vi "CmdExe.Command Line Output to Log text.vi"(11 "CmdLineOut":T1) -> (3 "Log Text":string)   [LabVIEW 2024]
uses:
  CmdExe.Command Line Output Info.ctl
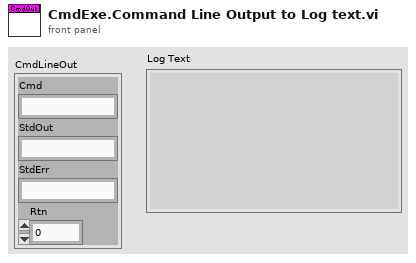
[diagram p1: front panel]
types:
  T1 = typedef "CmdExe.Command Line Output Info.ctl" = cluster{"Cmd":string, "StdOut":string, "StdErr":string, "Rtn":i32}
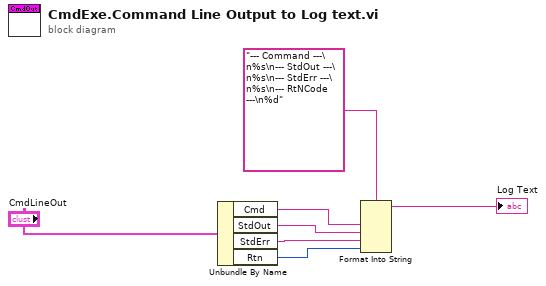
[diagram p0: block diagram]
diagram:
  n1 = Unbundle By Name("CmdLineOut") -> ("Cmd"=w5:string, "StdOut"=w4:string, "StdErr"=w3:string, "Rtn"=w2:i32)
  n2 = Format Into String(format string="--- Command ---\n%s\n--- StdOut ---\n%s\n--- StdErr ---\n%s\n--- RtNCode ---\n%d", w5, w4, w3, w2) -> (resulting string=→"Log Text":string)  [unwired: 2 in, 1 out]
